vi "qDIA.vi"(0 "System no.":i32=1 min=1 max=4 step=1, 2 "MeasureIDs to query":i32[](array[numeric]), 3 "All IDs?":bool, 5 "error in":errorcluster) -> (14 "Measured values":string[](array[string]), 19 "error out":errorcluster)   [LabVIEW 2020]
doc: "Returns diagnosis information. Use HDI?.vi to find out valid MeasureIDs and their meanings. \n\nE-870: If All ID's? = FALSE, only one MeasureID to query per command allowed."
panel:
  # "Get diagnosis information. User HDI?.vi to find out valid MeasureIDs and\ntheir meanings."
  # "Query"
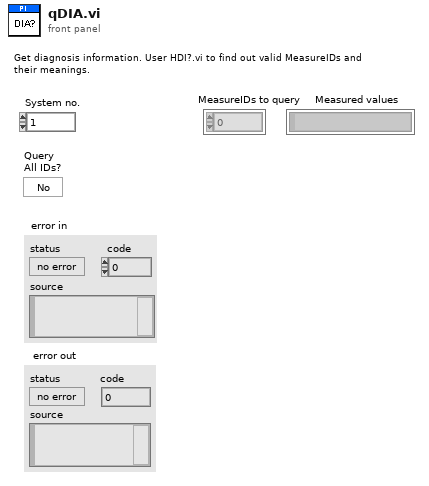
[diagram p1: front panel]
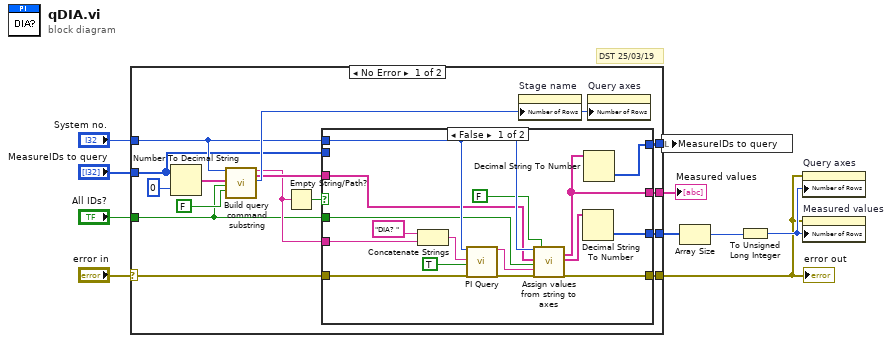
[diagram p0: block diagram]
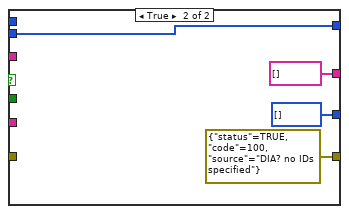
[diagram p2: hidden frame]
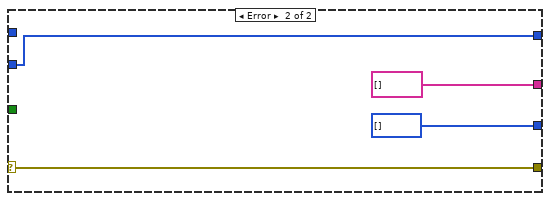
[diagram p3: hidden frame]
diagram:
  # "DST 25/03/19"
  n1 = case shown="No Error" "error in" {
    selector: "error in" -> [w15 w47]
    tunnel: "MeasureIDs to query" -> [w11 w46]
    tunnel: [w18 w47] -> w2
    tunnel: "System no." -> [w24 _]
    tunnel: "All IDs?" -> [w13 _]
    tunnel: [w23 string[] [] ("Strings")] -> w3
    tunnel: [w16 i32[] []] -> w7
    tunnel: [w12 w46] -> w1
    frame No Error {
      n2 = Number To Decimal String(number=w11, width (-)=i16 0) -> (decimal integer string=w20:string[])
      n3 = call "Build query command substring.vi"("System no."=w24, "Axes to query in"=w20, "Query\nAll axes?"=w13, "For all axes: use\nAxis identifier?"=FALSE ("Axis Identifier?")) -> ("Command substring"=w17:string, "Axes to query out"=w19:string[], "Number of rows"=w25:u32)  [unwired: 2 in, 11 out]
      n4 = Empty String/Path?(string/path=w17) -> (empty?=w14:bool)
      n5 = case shown="False" w14 {
        tunnel: w24 -> [w38 _]
        tunnel: w13 -> [w37 _]
        tunnel: [w27 string[] [] ("Strings")] -> w23
        tunnel: w19 -> [w36 _]
        tunnel: [w34 errorcluster {"status"=TRUE, "code"=100, "source"="DIA? no IDs specified"} ("error out")] -> w18
        tunnel: w17 -> [w30 _]
        tunnel: [w29 i32[] []] -> w16
        tunnel: w15 -> [w28 _]
        tunnel: [w26 w42] -> w12
        tunnel: w11 -> [_ w42]
        frame False {
          n6 = Concatenate Strings("DIA? ", w30) -> (w39:string)
          n7 = call "PI Query.vi"("System no."=w38, "String to send"=w39, "Attach termination char.?"=TRUE ("Attach Linefeed?"), "error in"=w28) -> ("String read"=w32:string, "error out"=w31:errorcluster)  [unwired: 3 in, 11 out]
          n8 = call "Assign values from string to axes.vi"("System no."=w38, "Queried axes"=w36, "All axes queried?"=w37, "Input String"=w32, "error in"=w31, "Axes related?"=FALSE) -> ("Strings"=w27:string[], "Queried axes out"=w33:string[], "error out"=w34:errorcluster)  [unwired: 3 in, 8 out]
          n9 = Decimal String To Number(string=w33) -> (number=w29:i32[])  [unwired: 3 out]
          n10 = Decimal String To Number(string=w27) -> (number=w26:i32[])  [unwired: 3 out]
        }
        frame True {
        }
      }
      n11 = property on="Stage name" class="Arr (strict)"("Number of Rows"=w25) -> ()  [unwired: 2 in, 2 out]
      n12 = property on="Query axes" class="Arr (strict)"("Number of Rows"=w25) -> ()  [unwired: 2 in, 2 out]
    }
    frame Error {
    }
  }
  "error out" <- w2
  "Measured values" <- w3
  n13 = local write "MeasureIDs to query"(w1) -> ()
  n14 = Array Size(array=w7) -> (size(s)=w6:i32)
  n15 = To Unsigned Long Integer(number=w6) -> (unsigned 32bit integer=w5:u32)
  n16 = property on="Query axes" class="Arr (strict)"(error in=w2, "Number of Rows"=w5) -> ()  [unwired: 1 in, 2 out]
  n17 = property on="Measured values" class="Arr (strict)"(error in=w2, "Number of Rows"=w5) -> ()  [unwired: 1 in, 2 out]
